vi "Get SMO Public API.vi"(8 "error in (no error)":errorcluster, 11 "Example Instrument in":refnum<class "ExampleInstrument.lvclass">) -> (0 "error out":errorcluster, 2 "Commands":string[](array[string]), 3 "Example Instrument out":refnum<class "ExampleInstrument.lvclass">)   [LabVIEW 2016, in "ExampleInstrument.lvclass"]
uses:
  ExampleInstrument.lvclass
  Typedefs/ExampleInstrument.Commands--Enum.ctl
  SMOs/Instrument/Instrument.lvclass
panel:
  in  "Commands":T1
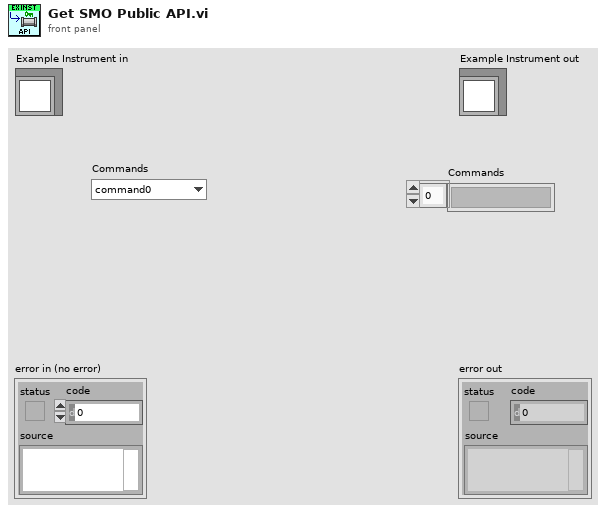
[diagram p1: front panel]
types:
  T1 = typedef "ExampleInstrument.lvclass/ExampleInstrument.Commands--Enum.ctl" = enum16{"command0", "command1", "command2"}
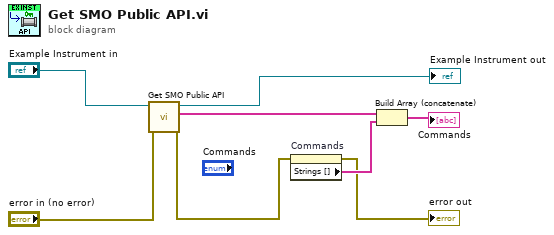
[diagram p0: block diagram]
diagram:
  n1 = call-parent "Get SMO Public API.vi"("error in (no error)"="error in (no error)", "Instrument in"="Example Instrument in") -> ("error out"=w2:errorcluster, "Commands"=w7:string[], "Instrument out"=→"Example Instrument out":refnum<class "ExampleInstrument.lvclass">)  [unwired: 7 in]
  n2 = property on="Commands" class="Enum (strict)"(error in=w2) -> (error out=→"error out":errorcluster, "Strings []"=w3:string[])  [unwired: 1 in, 1 out]
  n3 = Build Array (concatenate)(w7, w3) -> (→"Commands":string[])
